vi "StepRun.vi"(5 "EndTime":timestamp, 7 "StartTime":timestamp, 8 "error in":errorcluster, 11 "StepRun":refnum<class "StepRun.lvclass">) -> (0 "error out":errorcluster, 3 "Passed":bool)   [LabVIEW 2020]
uses:
  ProligentResultProcessor/StepRun/StepRun/StepRun.lvclass
  ProligentResultProcessor/StepRun/StepRun/SetStepName.vi
  ProligentResultProcessor/StepRun/StepRun/SetStepExecutionStatus.vi
  ProligentResultProcessor/StepRun/StepRun/SetStartDate.vi
  ProligentResultProcessor/StepRun/StepRun/SetEndDate.vi
  ProligentResultProcessor/StepRun/StepRun/SetStepRunId.vi
  ProligentResultProcessor/StepRun/StepRun/GetStepName.vi
  ProligentResultProcessor/StepRun/StepRun/GetStepExecutionStatus.vi
  ProligentResultProcessor/StepRun/StepRun/GetStartDate.vi
  ProligentResultProcessor/StepRun/StepRun/GetEndDate.vi
  ProligentResultProcessor/StepRun/StepRun/GetStepRunId.vi
  ProligentResultProcessor/StepRun/StepRun/GetMeasures.vi
  ProligentResultProcessor/StepRun/StepRun/GetCharacteristics.vi
  ProligentResultProcessor/StepRun/StepRun/GetDocuments.vi
  ProligentResultProcessor/StepRun/StepRun/GetFailureReferences.vi
  ProligentResultProcessor/StepRun/StepRun/GetCustomData.vi
  ProligentResultProcessor/Measure/Measure/Measure.lvclass
  ProligentResultProcessor/Model/Characteristic/Characteristic.lvclass
  ProligentResultProcessor/Model/Document/Document.lvclass
  ProligentResultProcessor/Failure/FailureReference/FailureReference.lvclass
  ProligentResultProcessor/Model/CustomData/CustomData.lvclass
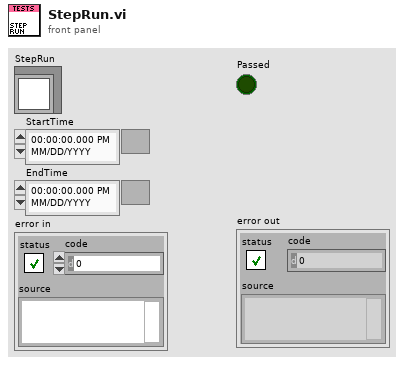
[diagram p1: front panel]
types:
  T1 = enum16{"PASS", "FAIL", "NOT_COMPLETED", "ABORTED"}
  T2 = typedef "ProligentResultProcessor.lvlib/ExecutionStatus.lvclass/Value.ctl" = enum16{"PASS", "FAIL", "NOT_COMPLETED", "ABORTED"}
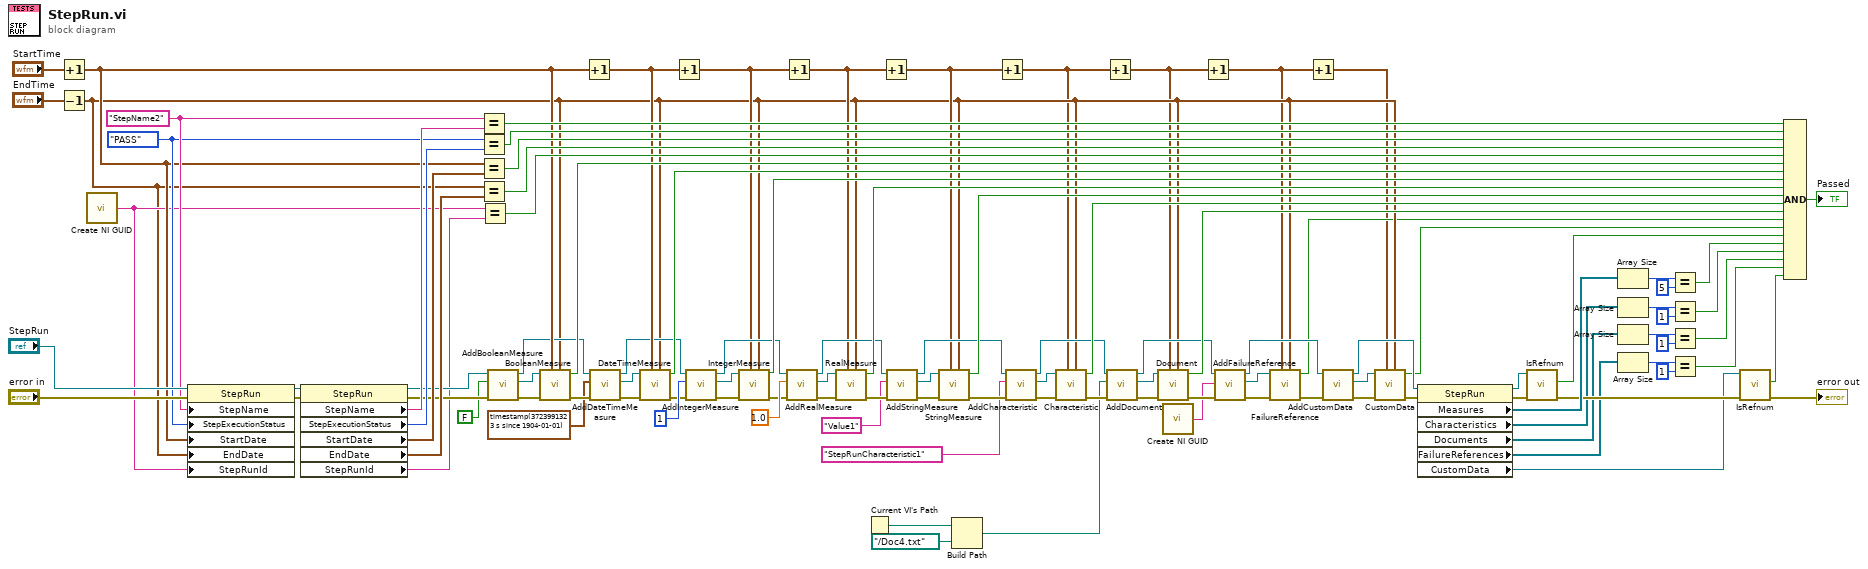
[diagram p0: block diagram]
diagram:
  w78 = T1."PASS" ("ProcessRunStatus")
  w89 = "StepName2"
  n1 = Increment(x="StartTime") -> (x+1=w56:timestamp)
  n2 = Decrement(x="EndTime") -> (x-1=w11:timestamp)
  n3 = call <vilib>:"Create NI GUID.vi"() -> ("NI GUID"=w29:string)
  n4 = property class="StepRun"(reference="StepRun", error in="error in", "StepName"=w89, "StepExecutionStatus"=w78, "StartDate"=w56, "EndDate"=w11, "StepRunId"=w29) -> (reference out=w95:refnum<class "StepRun.lvclass">, error out=w94:errorcluster)
  n5 = property class="StepRun"(reference=w95, error in=w94) -> (reference out=w88:refnum<class "StepRun.lvclass">, error out=w87:errorcluster, "StepName"=w93:string, "StepExecutionStatus"=w92:T2, "StartDate"=w91:timestamp, "EndDate"=w90:timestamp, "StepRunId"=w30:string)
  n6 = Equal?(x=w89, y=w93) -> (x = y?=w108:bool)
  n7 = Equal?(x=w78, y=w92) -> (x = y?=w107:bool)
  n8 = Equal?(x=w56, y=w91) -> (x = y?=w106:bool)
  n9 = Equal?(x=w11, y=w90) -> (x = y?=w110:bool)
  n10 = Equal?(x=w29, y=w30) -> (x = y?=w109:bool)
  n11 = call "AddBooleanMeasure.vi"("error in"=w87, "Value"=FALSE, "StepRun in"=w88) -> ("error out"=w75:errorcluster, "BooleanMeasure"=w76:refnum<class "BooleanMeasure.lvclass">, "StepRun out"=w53:refnum<class "StepRun.lvclass">)  [unwired: 6 in]
  n12 = call "BooleanMeasure.vi"("EndTime"=w11, "StartTime"=w56, "error in"=w75, "BooleanMeasure"=w76) -> ("error out"=w63:errorcluster, "Passed"=w104:bool)  [unwired: 6 in]
  n13 = Increment(x=w56) -> (x+1=w55:timestamp)
  n14 = call "AddDateTimeMeasure.vi"("error in"=w63, "Value"=timestamp(3723991323.456 s since 1904-01-01), "StepRun in"=w53) -> ("error out"=w58:errorcluster, "RealMeasure"=w54:refnum<class "DateTimeMeasure.lvclass">, "StepRun out"=w52:refnum<class "StepRun.lvclass">)  [unwired: 6 in]
  n15 = call "DateTimeMeasure.vi"("EndTime"=w11, "StartTime"=w55, "error in"=w58, "DateTimeMeasure"=w54) -> ("error out"=w57:errorcluster, "Passed"=w100:bool)  [unwired: 6 in]
  n16 = Increment(x=w55) -> (x+1=w64:timestamp)
  n17 = call "AddIntegerMeasure.vi"("error in"=w57, "Value"=i64 1, "StepRun in"=w52) -> ("error out"=w68:errorcluster, "RealMeasure"=w67:refnum<class "IntegerMeasure.lvclass">, "StepRun out"=w66:refnum<class "StepRun.lvclass">)  [unwired: 6 in]
  n18 = call "IntegerMeasure.vi"("EndTime"=w11, "StartTime"=w64, "error in"=w68, "IntegerlMeasure"=w67) -> ("error out"=w65:errorcluster, "Passed"=w102:bool)  [unwired: 6 in]
  n19 = Increment(x=w64) -> (x+1=w49:timestamp)
  n20 = call "AddRealMeasure.vi"("error in"=w65, "Value"=1.0, "StepRun in"=w66) -> ("error out"=w72:errorcluster, "RealMeasure"=w71:refnum<class "RealMeasure.lvclass">, "StepRun out"=w59:refnum<class "StepRun.lvclass">)  [unwired: 6 in]
  n21 = call "RealMeasure.vi"("EndTime"=w11, "StartTime"=w49, "error in"=w72, "RealMeasure"=w71) -> ("error out"=w62:errorcluster, "Passed"=w103:bool)  [unwired: 6 in]
  n22 = Current VI's Path() -> (path=w3:path)
  n23 = Increment(x=w49) -> (x+1=w12:timestamp)
  n24 = call "AddStringMeasure.vi"("error in"=w62, "Value"="Value1", "StepRun in"=w59) -> ("error out"=w50:errorcluster, "StringMeasure"=w51:refnum<class "StringMeasure.lvclass">, "StepRun out"=w35:refnum<class "StepRun.lvclass">)  [unwired: 6 in]
  n25 = call "StringMeasure.vi"("EndTime"=w11, "StartTime"=w12, "error in"=w50, "StringMeasure"=w51) -> ("error out"=w39:errorcluster, "Passed"=w101:bool)  [unwired: 6 in]
  n26 = Build Path(base path=w3, name or relative path=path "../Doc4.txt" ("FilePath")) -> (appended path=w1:path)
  n27 = Increment(x=w12) -> (x+1=w7:timestamp)
  n28 = call "AddCharacteristic.vi"("error in"=w39, "FullName"="StepRunCharacteristic1", "StepRun in"=w35) -> ("error out"=w38:errorcluster, "Characteristic"=w36:refnum<class "Characteristic.lvclass">, "StepRun out"=w32:refnum<class "StepRun.lvclass">)  [unwired: 6 in]
  n29 = call "Characteristic.vi"("EndTime"=w11, "StartTime"=w7, "error in (no error)"=w38, "Characteristic in"=w36) -> ("error out"=w37:errorcluster, "Passed"=w99:bool)  [unwired: 6 in]
  n30 = Increment(x=w7) -> (x+1=w6:timestamp)
  n31 = call "AddDocument.vi"("error in"=w37, "FilePath"=w1, "StepRun in"=w32) -> ("error out"=w33:errorcluster, "Document"=w31:refnum<class "Document.lvclass">, "StepRun out"=w26:refnum<class "StepRun.lvclass">)  [unwired: 6 in]
  n32 = call "Document.vi"("EndTime"=w11, "StartTime"=w6, "error in (no error)"=w33, "Characteristic in"=w31) -> ("error out"=w28:errorcluster, "Passed"=w98:bool)  [unwired: 6 in]
  n33 = call <vilib>:"Create NI GUID.vi"() -> ("NI GUID"=w10:string)
  n34 = Increment(x=w6) -> (x+1=w5:timestamp)
  n35 = call "AddFailureReference.vi"("error in"=w28, "Id"=w10, "StepRun in"=w26) -> ("error out"=w27:errorcluster, "FailureReference"=w24:refnum<class "FailureReference.lvclass">, "StepRun out"=w16:refnum<class "StepRun.lvclass">)  [unwired: 6 in]
  n36 = call "FailureReference.vi"("EndTime"=w11, "StartTime"=w5, "error in"=w27, "Defect"=w24) -> ("error out"=w25:errorcluster, "Passed"=w9:bool)  [unwired: 6 in]
  n37 = Increment(x=w5) -> (x+1=w4:timestamp)
  n38 = call "AddCustomData.vi"("error in (no error)"=w25, "StepRun in"=w16) -> ("error out"=w17:errorcluster, "CustomData"=w13:refnum<class "CustomData.lvclass">, "StepRun out"=w15:refnum<class "StepRun.lvclass">)  [unwired: 7 in]
  n39 = call "CustomData.vi"("EndTime"=w11, "StartTime"=w4, "error in"=w17, "CustomData"=w13) -> ("error out"=w14:errorcluster, "Passed"=w8:bool)  [unwired: 6 in]
  n40 = property class="StepRun"(reference=w15, error in=w14) -> (reference out=w73:refnum<class "StepRun.lvclass">, error out=w83:errorcluster, "Measures"=w84:refnum<class "Measure.lvclass">[], "Characteristics"=w23:refnum<class "Characteristic.lvclass">[], "Documents"=w22:refnum<class "Document.lvclass">[], "FailureReferences"=w21:refnum<class "FailureReference.lvclass">[], "CustomData"=w19:refnum<class "CustomData.lvclass">)
  n41 = call "IsRefnum.vi"("error in"=w83, "StepRun in"=w73) -> ("error out"=w74:errorcluster, "IsRefnum"=w105:bool)  [unwired: 7 in, 1 out]
  n42 = Array Size(array=w84) -> (size(s)=w86:i32)
  n43 = Array Size(array=w23) -> (size(s)=w47:i32)
  n44 = Array Size(array=w22) -> (size(s)=w46:i32)
  n45 = Array Size(array=w21) -> (size(s)=w43:i32)
  n46 = Equal?(x=w86, y=5) -> (x = y?=w82:bool)
  n47 = Equal?(x=w47, y=1) -> (x = y?=w42:bool)
  n48 = Equal?(x=w46, y=1) -> (x = y?=w41:bool)
  n49 = Equal?(x=w43, y=1) -> (x = y?=w40:bool)
  n50 = call "IsRefnum.vi"("error in"=w74, "CustomDataType in"=w19) -> ("error out"=→"error out":errorcluster, "IsRefnum"=w18:bool)  [unwired: 7 in, 1 out]
  n51 = Compound Arithmetic op=AND(w108, w107, w106, w110, w109, w104, w100, w102, w103, w101, w99, w98, w9, w8, w105, w82, w42, w41, w40, w18) -> (→"Passed":bool)
